vi "Stop All Terminals.vi"(8 "error in (no error)":errorcluster, 11 "Manager in":refnum<class "Manager.lvclass">) -> (0 "error out":errorcluster, 3 "Manager out":refnum<class "Manager.lvclass">)   [LabVIEW 2025, in "Manager.lvlib" / "Manager.lvclass"]
uses:
  Manager.lvclass
  Manager.lvclass/Manager.ctl
  <vilib>/ActorFramework/Stop Msg/Stop Msg.lvclass
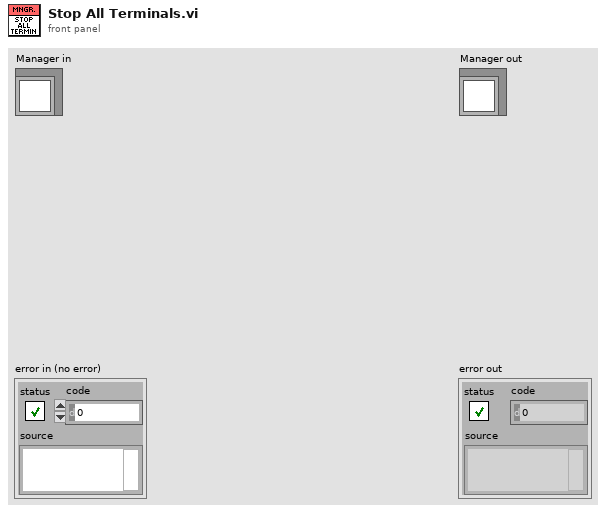
[diagram p1: front panel]
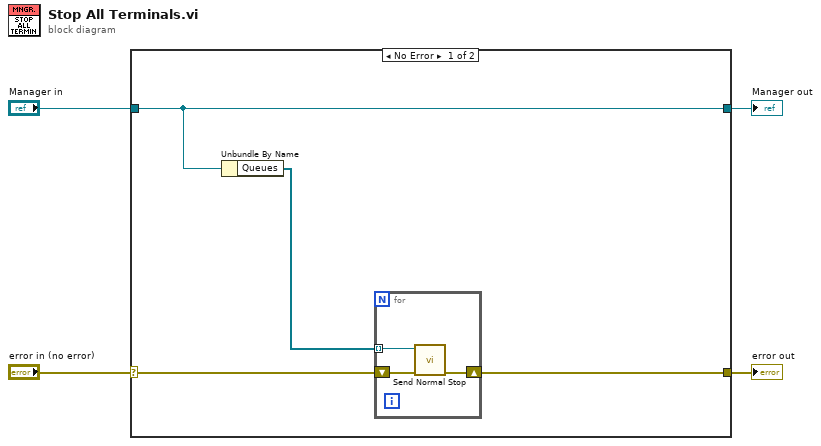
[diagram p0: block diagram]
diagram:
  n1 = case shown="No Error" "error in (no error)" {
    selector: "error in (no error)" -> [w8 w13]
    tunnel: [w7 w13] -> w3
    tunnel: [w6 w12] -> w1
    tunnel: "Manager in" -> [w6 w12]
    frame No Error {
      n2 = Unbundle By Name(w6) -> ("Queues"=w5:refnum<class "Message Enqueuer.lvclass">[])
      n3 = for {
        shift-right: [w10] -> w7
        shift-left: w8 -> [w11]
        tunnel: w5 -> [w9] mode=indexing
        n4 = call <vilib>:"Send Normal Stop.vi"("error in (no error)"=w11, "Message Enqueuer"=w9) -> ("error out"=w10:errorcluster)  [unwired: 9 in]
      }
    }
    frame Error {
    }
  }
  "error out" <- w3
  "Manager out" <- w1
